vi "Set Taps.vi"(8 "error in (no error)":errorcluster, 10 "Taps":i32(ring) items=["SingleTap", "DualTap", "QuadTap"], 11 "TLCamera reference in":refnum<k24>) -> (0 "error out":errorcluster, 3 "TLCamera reference out":refnum<k24>)   [LabVIEW 2019]
uses:
  C:/Users/jleeman/git_repos/CAxis_Machine/C-Axis LabView Controller/Library_X64/Thorlabs.TSI.TLCameraInterfaces.dll
  Library_X64/Thorlabs.TSI.TLCameraInterfaces.dll
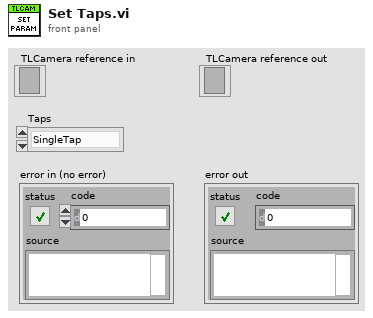
[diagram p1: front panel]
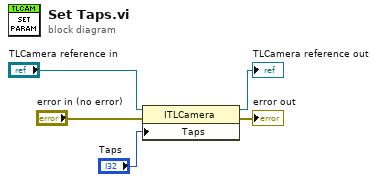
[diagram p0: block diagram]
diagram:
  n1 = property class="ITLCamera"(reference="TLCamera reference in", error in="error in (no error)", "Taps"="Taps") -> (reference out=→"TLCamera reference out":refnum<k24>, error out=→"error out":errorcluster)
